vi "Construct MVA Comms Objects.vi"(0 "MVA Project Reference":refnum<vi>) -> (4 "MVA Comms VIs":refnum<class "MVA Comms VI Instance.lvclass">[](array[class]))   [LabVIEW 2019, in "MVA Message Mapper.lvlib"]
uses:
  <vilib>/gpm_packages/@cs/Bus-message-mapper/Source/MVA Message Mapper.lvlib
  <vilib>/gpm_packages/@cs/Bus-message-mapper/Source/support/MVA Comms/MVA Comms VI Instance.lvclass
  <vilib>/gpm_packages/@cs/Bus-message-mapper/Source/support/Bind to Control Ref/Bind To Control Ref.lvclass
  C:/Program Files/National Instruments/LabVIEW 2019/vi.lib/gpm_packages/@cs/Bus-message-mapper/Source/support/MVA Comms/MVA Comms VI Instance.lvclass
  <vilib>/gpm_packages/@cs/Bus-message-mapper/Source/support/MVA Comms/MVA Comms VI Instance.lvclass/MVA Comms VI Instance.ctl
  <vilib>/gpm_packages/@cs/Bus-message-mapper/Source/support/MVA Comms/Accessors/Write Project Reference.vi
  <vilib>/gpm_packages/@cs/Bus-message-mapper/Source/support/MVA Comms/Accessors/Write MVA Coms VI Name.vi
  <vilib>/gpm_packages/@cs/Bus-message-mapper/Source/support/MVA Comms/Accessors/Write Broadcaster.vi
  <vilib>/gpm_packages/@cs/Bus-message-mapper/Source/support/MVA Comms/Accessors/Write Datum Name Terminal.vi
  <vilib>/gpm_packages/@cs/Bus-message-mapper/Source/support/MVA Comms/Accessors/Write Datum Value Terminal.vi
  <vilib>/gpm_packages/@cs/Bus-message-mapper/Source/support/MVA Comms/Accessors/Write MVA Object In Terminal.vi
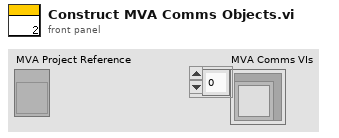
[diagram p1: front panel]
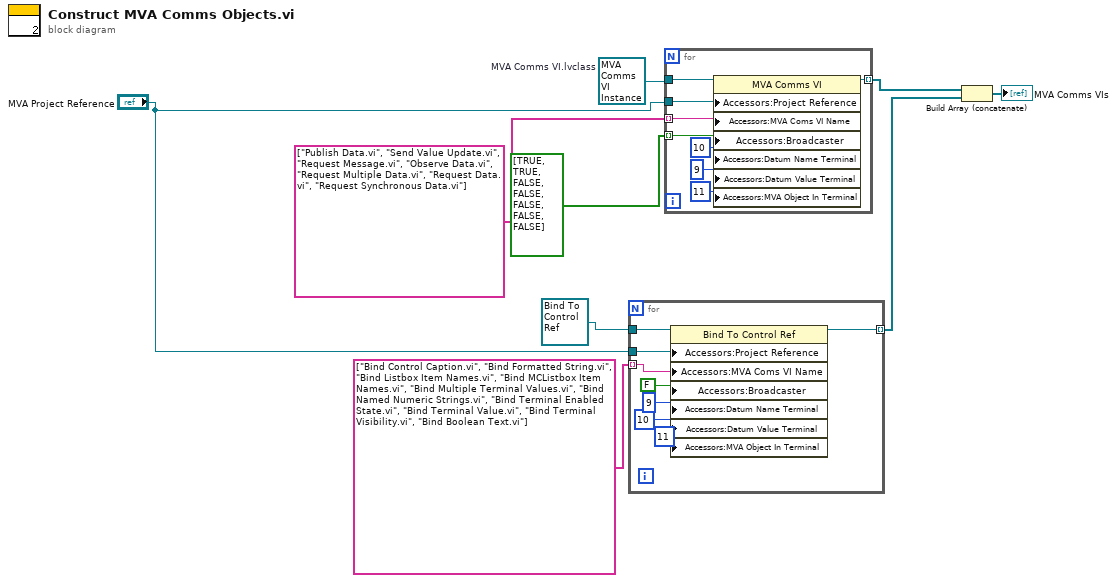
[diagram p0: block diagram]
diagram:
  w3 = refnum<class "MVA Comms VI Instance.lvclass"> refnum  # MVA Comms VI.lvclass
  n1 = for {
    tunnel: "MVA Project Reference" -> [w14]
    tunnel: string[] ["Bind Control Caption.vi", "Bind Formatted String.vi", "Bind Listbox Item Names.vi", "Bind MCListbox Item Names.vi", "Bind Multiple Terminal Values.vi", "Bind Named Numeric Strings.vi", "Bind Terminal Enabled State.vi", "Bind Terminal Value.vi", "Bind Terminal Visibility.vi", "Bind Boolean Text.vi"] ("array") -> [w11] mode=indexing
    tunnel: refnum<class "Bind To Control Ref.lvclass"> refnum ("MVA Message Mapper.lvlib:Bind To Control Ref") -> [w12]
    tunnel: [w13] -> w5 mode=indexing
    n2 = property on="Property Node" class="Bind To Control Ref"(reference=w12, "Accessors:Project Reference"=w14, "Accessors:MVA Coms VI Name"=w11, "Accessors:Broadcaster"=FALSE ("Broadcaster"), "Accessors:Datum Name Terminal"=9 ("Datum Name Terminal"), "Accessors:Datum Value Terminal"=10 ("Datum Value Terminal"), "Accessors:MVA Object In Terminal"=11 ("MVA Object In Terminal")) -> (reference out=w13:refnum<class "Bind To Control Ref.lvclass">)  [unwired: 1 in, 1 out]
  }
  n3 = for {
    tunnel: [w25] -> w6 mode=indexing
    tunnel: w3 -> [w24]
    tunnel: bool[] [TRUE, TRUE, FALSE, FALSE, FALSE, FALSE, FALSE] -> [w23] mode=indexing
    tunnel: string[] ["Publish Data.vi", "Send Value Update.vi", "Request Message.vi", "Observe Data.vi", "Request Multiple Data.vi", "Request Data.vi", "Request Synchronous Data.vi"] -> [w22] mode=indexing
    tunnel: "MVA Project Reference" -> [w21]
    n4 = property class="MVA Comms VI"(reference=w24, "Accessors:Project Reference"=w21, "Accessors:MVA Coms VI Name"=w22, "Accessors:Broadcaster"=w23, "Accessors:Datum Name Terminal"=10 ("Datum Name Terminal"), "Accessors:Datum Value Terminal"=9 ("Datum Value Terminal"), "Accessors:MVA Object In Terminal"=11 ("MVA Object In Terminal")) -> (reference out=w25:refnum<class "MVA Comms VI Instance.lvclass">)  [unwired: 1 in, 1 out]
  }
  n5 = Build Array (concatenate)(w6, w5) -> (→"MVA Comms VIs":refnum<class "MVA Comms VI Instance.lvclass">[])
